vi "6.vi"   [LabVIEW 2017]
uses:
  <vilib>/Utility/file.llb/Write Delimited Spreadsheet (string).vi
  <vilib>/Utility/file.llb/Write Delimited Spreadsheet (DBL).vi
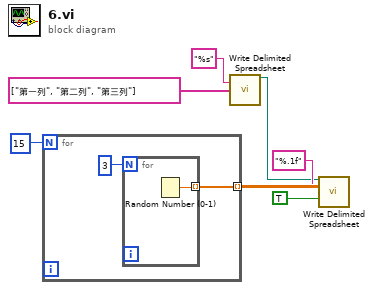
[diagram p0: block diagram]
diagram:
  n1 = for {
    N: 15 -> [_]
    tunnel: [w8] -> w6 mode=indexing
    n2 = for {
      N: 3 -> [_]
      tunnel: [w10] -> w8 mode=indexing
      n3 = Random Number (0-1)() -> (number: 0 to 1=w10:dbl)
    }
  }
  n4 = call-poly <vilib>:"Write Delimited Spreadsheet.vi"("format (%s)"="%s", "1D data"=string[] ["第一列", "第二列", "第三列"]) -> ("new file path (Not A Path if cancelled)"=w2:path)  [unwired: 12 in, 1 out]
  n5 = call-poly <vilib>:"Write Delimited Spreadsheet.vi"("file path (dialog if empty)"=w2, "format (%.3f)"="%.1f", "2D data"=w6, "append to file? (new file:F)"=TRUE) -> ()  [unwired: 10 in, 2 out]
